vi "Get Window Text_KT.vi"(6 "nMaxCount":i32, 8 "Name (Byte)":string, 9 "hWnd":u32) -> (2 "Name":string, 3 "hWnd dup":u32)   [LabVIEW 2017, in "KTools.lvlib"]
doc: "<------------Get Window Text-------------->\nReturns window name of the given hWnd. \nnMaxCount: This is the maximum length of the window name expected."
uses:
  KTools.lvlib
  user32.dll
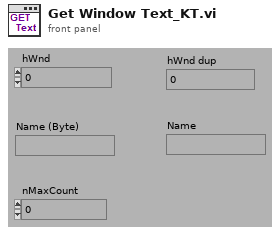
[diagram p1: front panel]
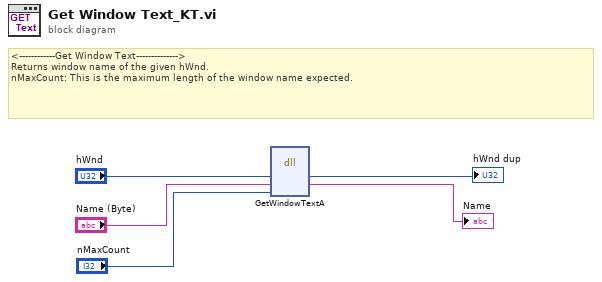
[diagram p0: block diagram]
diagram:
  # "<------------Get Window Text-------------->\nReturns window name of the given hWnd. \nnMaxCount: This is the maximum length of the window name expected."
  n1 = dll-call lib="user32.dll" fn="GetWindowTextA" ("GetActiveWindow")("hWnd"="hWnd", "lpString"="Name (Byte)", "nMaxCount"="nMaxCount") -> ("hWnd"=→"hWnd dup":u32, "lpString"=→"Name":string)  [unwired: 5 in, 2 out]
